vi "CreateCommands.vi"   [LabVIEW 2014]
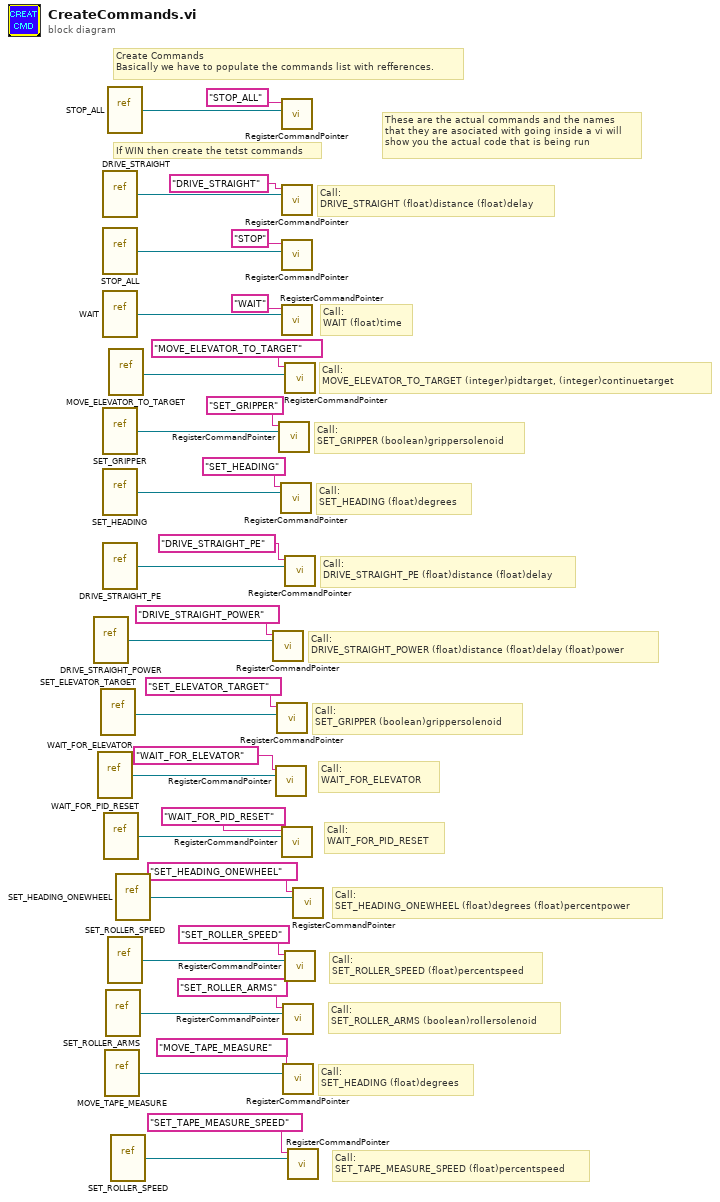
[diagram p0: block diagram]
diagram:
  # "Call:\nSET_TAPE_MEASURE_SPEED (float)percentspeed"
  # "Call:\nSET_HEADING (float)degrees"
  # "Call:\nSET_ROLLER_SPEED (float)percentspeed"
  # "Call:\nSET_ROLLER_ARMS (boolean)rollersolenoid"
  # "Call:\nSET_HEADING_ONEWHEEL (float)degrees (float)percentpower"
  # "Call:\nMOVE_ELEVATOR_TO_TARGET (integer)pidtarget, (integer)continuetarget"
  # "Call:\nWAIT_FOR_PID_RESET"
  # "Call:\nDRIVE_STRAIGHT_POWER (float)distance (float)delay (float)power"
  # "Call:\nWAIT_FOR_ELEVATOR"
  # "Call:\nSET_GRIPPER (boolean)grippersolenoid"
  # "Call:\nDRIVE_STRAIGHT_PE (float)distance (float)delay"
  # "Call:\nSET_HEADING (float)degrees"
  # "Call:\nSET_GRIPPER (boolean)grippersolenoid"
  # "Call:\nDRIVE_STRAIGHT (float)distance (float)delay"
  # "These are the actual commands and the names \nthat they are asociated with going inside a vi will\nshow you the actual code that is being run"
  # "Call:\nWAIT (float)time"
  # "If WIN then create the tetst commands"
  # "Create Commands\nBasically we have to populate the commands list with refferences."
  n1 = vi-ref "DRIVE_STRAIGHT_POWER.vi"() -> (w13:refnum<vi>)
  n2 = vi-ref "WAIT_FOR_ELEVATOR.vi"() -> (w18:refnum<vi>)
  n3 = vi-ref "SET_ELEVATOR_TARGET.vi"() -> (w19:refnum<vi>)
  n4 = vi-ref "DRIVE_STRAIGHT.vi"() -> (w31:refnum<vi>)
  n5 = vi-ref "STOP_ALL.vi"() -> (w28:refnum<vi>)
  n6 = vi-ref "WAIT.vi"() -> (w29:refnum<vi>)
  n7 = vi-ref "SET_GRIPPER.vi"() -> (w25:refnum<vi>)
  n8 = vi-ref "SET_HEADING.vi"() -> (w23:refnum<vi>)
  n9 = vi-ref "DRIVE_STRAIGHT_PE.vi"() -> (w21:refnum<vi>)
  n10 = vi-ref "WAIT_FOR_PID_RESET.vi"() -> (w12:refnum<vi>)
  n11 = vi-ref "MOVE_TAPE_MEASURE.vi"() -> (w4:refnum<vi>)
  n12 = vi-ref "SET_ROLLER_ARMS.vi"() -> (w5:refnum<vi>)
  n13 = vi-ref "STOP_ALL.vi"() -> (w33:refnum<vi>)
  n14 = vi-ref "SET_ROLLER_SPEED.vi"() -> (w7:refnum<vi>)
  n15 = vi-ref "MOVE_ELEVATOR_TO_TARGET.vi"() -> (w15:refnum<vi>)
  n16 = vi-ref "SET_ROLLER_SPEED.vi"() -> (w1:refnum<vi>)
  n17 = vi-ref "SET_HEADING_ONEWHEEL.vi"() -> (w9:refnum<vi>)
  n18 = call "RegisterCommandPointer.vi"("Strict-Typed VI Refnum"=w13, "Name"="DRIVE_STRAIGHT_POWER") -> ()  [unwired: 10 in]
  n19 = call "RegisterCommandPointer.vi"("Strict-Typed VI Refnum"=w18, "Name"="WAIT_FOR_ELEVATOR") -> ()  [unwired: 10 in]
  n20 = call "RegisterCommandPointer.vi"("Strict-Typed VI Refnum"=w19, "Name"="SET_ELEVATOR_TARGET") -> ()  [unwired: 10 in]
  n21 = call "RegisterCommandPointer.vi"("Strict-Typed VI Refnum"=w25, "Name"="SET_GRIPPER") -> ()  [unwired: 10 in]
  n22 = call "RegisterCommandPointer.vi"("Strict-Typed VI Refnum"=w23, "Name"="SET_HEADING") -> ()  [unwired: 10 in]
  n23 = call "RegisterCommandPointer.vi"("Strict-Typed VI Refnum"=w33, "Name"="STOP_ALL") -> ()  [unwired: 10 in]
  n24 = call "RegisterCommandPointer.vi"("Strict-Typed VI Refnum"=w31, "Name"="DRIVE_STRAIGHT") -> ()  [unwired: 10 in]
  n25 = call "RegisterCommandPointer.vi"("Strict-Typed VI Refnum"=w28, "Name"="STOP") -> ()  [unwired: 10 in]
  n26 = call "RegisterCommandPointer.vi"("Strict-Typed VI Refnum"=w29, "Name"="WAIT") -> ()  [unwired: 10 in]
  n27 = call "RegisterCommandPointer.vi"("Strict-Typed VI Refnum"=w12, "Name"="WAIT_FOR_PID_RESET") -> ()  [unwired: 10 in]
  n28 = call "RegisterCommandPointer.vi"("Strict-Typed VI Refnum"=w5, "Name"="SET_ROLLER_ARMS") -> ()  [unwired: 10 in]
  n29 = call "RegisterCommandPointer.vi"("Strict-Typed VI Refnum"=w4, "Name"="MOVE_TAPE_MEASURE") -> ()  [unwired: 10 in]
  n30 = call "RegisterCommandPointer.vi"("Strict-Typed VI Refnum"=w15, "Name"="MOVE_ELEVATOR_TO_TARGET") -> ()  [unwired: 10 in]
  n31 = call "RegisterCommandPointer.vi"("Strict-Typed VI Refnum"=w21, "Name"="DRIVE_STRAIGHT_PE") -> ()  [unwired: 10 in]
  n32 = call "RegisterCommandPointer.vi"("Strict-Typed VI Refnum"=w7, "Name"="SET_ROLLER_SPEED") -> ()  [unwired: 10 in]
  n33 = call "RegisterCommandPointer.vi"("Strict-Typed VI Refnum"=w1, "Name"="SET_TAPE_MEASURE_SPEED") -> ()  [unwired: 10 in]
  n34 = call "RegisterCommandPointer.vi"("Strict-Typed VI Refnum"=w9, "Name"="SET_HEADING_ONEWHEEL") -> ()  [unwired: 10 in]
